vi "Actor Core.vi"(8 "error in":errorcluster, 11 "Elevator Controller in":refnum<class "Sim Display Console Actor.lvclass">) -> (0 "error out":errorcluster, 3 "Actor out":refnum<class "Actor.lvclass">)   [LabVIEW 2019, in "Simulated Display Console Actor.lvlib" / "Sim Display Console Actor.lvclass"]
doc: "(<B>Filename</B>: Actor Framework.lvlib:Actor.lvclass:Actor Core.vi)\n\nReceives messages to the actor, reacts to them, and initiates any error handling that may shut the actor down.\n\nDescendant classes may override this VI to append parallel tasks for the actor to complete while it handles messages. Overrides use the Call Parent Method node."
uses:
  Sim Display Console Actor.lvclass
  <vilib>/ActorFramework/Stop Msg/Stop Msg.lvclass
  <vilib>/ActorFramework/Actor/Actor.lvclass
  C:/Workspace/CLA/Elevator AF 2nd/Dsiplay Console Actor/Dsiplay Console Actor/Dsiplay Console Actor.lvclass
  C:/Program Files (x86)/National Instruments/LabVIEW 2019/vi.lib/ActorFramework/Actor/Actor.lvclass
  Dsiplay Console Actor/Dsiplay Console Actor/Dsiplay Console Actor.lvclass
  Sim Display Console Actor Messages/Write Elevator Direction Msg/Write Elevator Direction Msg.lvclass
  Elevator Direction.ctl
  Sim Display Console Actor Messages/Write Elevator Location Msg/Write Elevator Location Msg.lvclass
  Floor -Enum.ctl
panel:
  out "Elevator Location":T1
  out "Emergency":bool
  out "Door Open":bool
  out "Timing":dbl
  out "Elevator Direction":T2
  # "[Covers: UI3] \n[Covers: UI3A] \n[Covers: UI3A1] \n[Covers: UI3A2] \n[Covers: UI3B] \n[Covers: UI3C] \n[Covers: UI3D] \n[Covers: UI3D1] \n[Covers: UI3D2] \n[Covers: UI3E]"
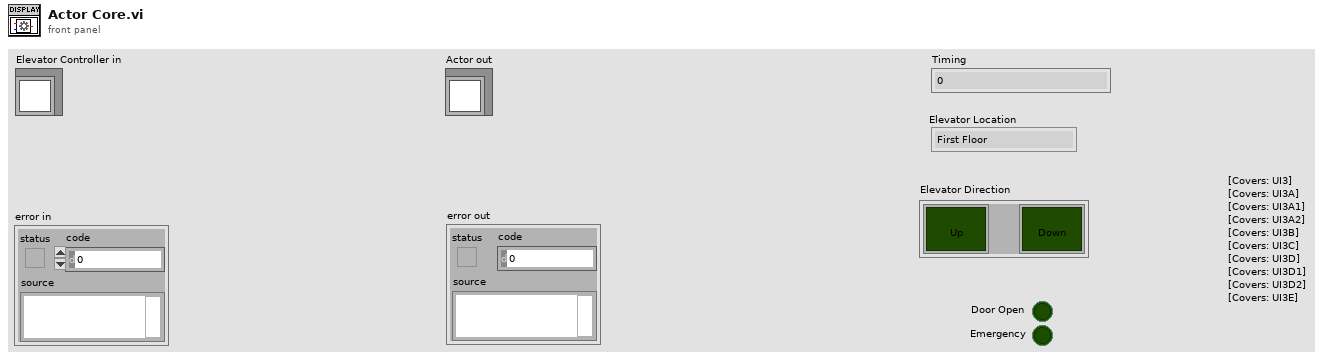
[diagram p1: front panel]
types:
  T1 = typedef "Simulated Display Console Actor.lvlib/Sim Display Console Actor.lvclass/Floor -Enum.ctl" = enum16{"First Floor", "Send Floor", "Third Floor", "Fourth Floor"}
  T2 = typedef "Simulated Display Console Actor.lvlib/Sim Display Console Actor.lvclass/Elevator Direction.ctl" = cluster{"Up":bool, "Down":bool}
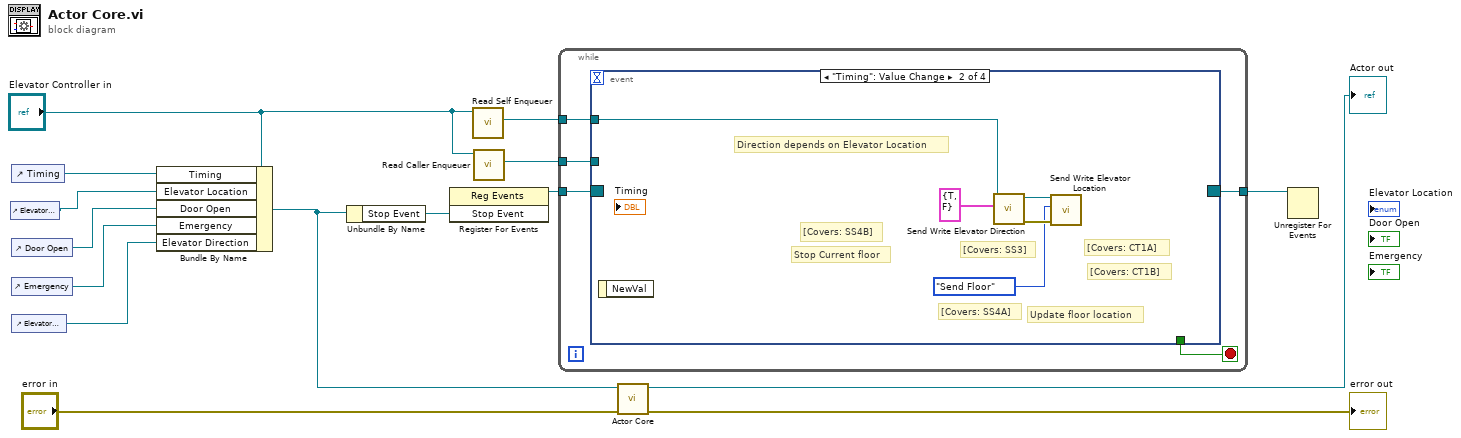
[diagram p0: block diagram]
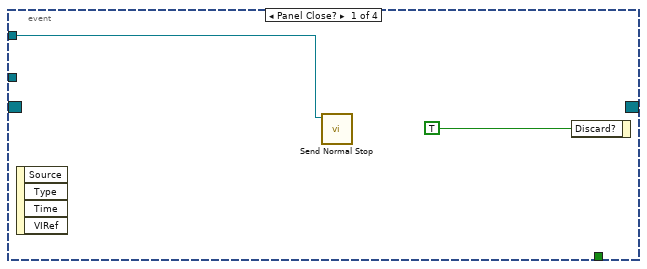
[diagram p2: hidden frame]
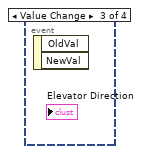
[diagram p3: hidden frame]
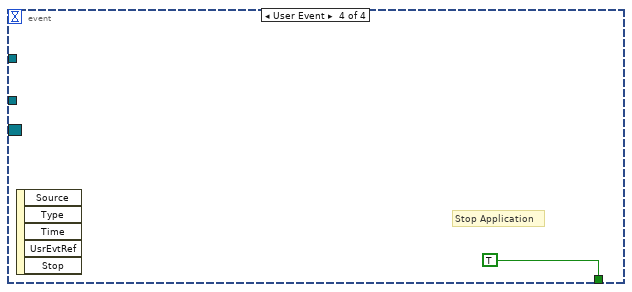
[diagram p4: hidden frame]
diagram:
  n1 = control-ref of="Elevator Location"() -> (w1:refnum<vi>)
  n2 = control-ref of="Timing"() -> (w5:refnum<vi>)
  n3 = control-ref of="Door Open"() -> (w4:refnum<vi>)
  n4 = control-ref of="Emergency"() -> (w3:refnum<vi>)
  n5 = control-ref of="Elevator Direction"() -> (w2:refnum<vi>)
  n6 = Bundle By Name(cluster="Elevator Controller in", "Timing"=w5, "Elevator Location"=w1, "Door Open"=w4, "Emergency"=w3, "Elevator Direction"=w2) -> (w6:refnum<class "Sim Display Console Actor.lvclass">)
  n7 = Unbundle By Name(w6) -> ("Stop Event"=w12:refnum<user-event>)
  n8 = register-events(w12) -> (reference out=w11:refnum<event-registration>)  [unwired: 2 in, 1 out]
  n9 = call <vilib>:"Read Self Enqueuer.vi"("Actor"="Elevator Controller in") -> ("Self Enqueuer"=w9:refnum<class "Message Enqueuer.lvclass">)  [unwired: 10 in]
  n10 = call <vilib>:"Read Caller Enqueuer.vi"("Actor"="Elevator Controller in") -> ("Caller Enqueuer"=w8:refnum<class "Message Enqueuer.lvclass">)  [unwired: 10 in]
  n11 = while {
    tunnel: w11 -> [w19]
    tunnel: [w18] -> w10
    tunnel: w9 -> [w17]
    tunnel: w8 -> [w16]
    stop <- w20 stop-if-true
    n12 = event shown="[1] \"Timing\": Value Change" {
      selector: w19 -> [_ _ _ _]
      dyn-events: [_ _ _ _] -> w18
      timeout: _ -> [_ _ _ _]
      tunnel: [_ _ _ TRUE] -> w20
      tunnel: w17 -> [w21 w26 _ _]
      tunnel: w16 -> [_ _ _ _]
      event Panel Close? {
        n13 = event-data() -> ()  [unwired: 1 in, 4 out]
        n14 = call <vilib>:"Send Normal Stop.vi"("Message Enqueuer"=w21) -> ()  [unwired: 10 in, 1 out]
        n15 = event-data("Discard?"=TRUE) -> ()  [unwired: 1 in, 1 out]
      }
      event "Timing": Value Change {
        # "[Covers: CT1B]"
        # "[Covers: CT1A]"
        # "Update floor location"
        # "[Covers: SS4B]"
        # "[Covers: SS4A]"
        # "Stop Current floor"
        # "[Covers: SS3]"
        # "Direction depends on Elevator Location"
        n16 = event-data() -> ()  [unwired: 1 in, 1 out]
        n17 = call "Send Write Elevator Direction.vi"("Elevator Direction"=T2 {"Up"=TRUE, "Down"=FALSE}, "Message Enqueuer"=w26) -> ("error out"=w24:errorcluster, "Message Enqueuer out"=w25:refnum<class "Message Enqueuer.lvclass">)  [unwired: 8 in]
        n18 = call "Send Write Elevator Location.vi"("error in (no error)"=w24, "Elevator Location"=Floor_-Enum."Send Floor", "Message Enqueuer"=w25) -> ()  [unwired: 7 in, 2 out]
      }
      event Value Change {
        n19 = event-data() -> ()  [unwired: 1 in, 2 out]
      }
      event User Event {
        # "Stop Application"
        n20 = event-data() -> ()  [unwired: 1 in, 5 out]
      }
    }
  }
  n21 = call-parent "Actor Core.vi"("error in"="error in", "Actor in"=w6) -> ("error out"=→"error out":errorcluster, "Actor out"=→"Actor out":refnum<class "Actor.lvclass">)  [unwired: 8 in]
  n22 = Unregister For Events(event registration refnum=w10) -> ()  [unwired: 1 in, 1 out]
